vi "Get RGB Pixels Values.vi"(9 "I_Number of columns":i16, 10 "I_Number of rows":i16, 11 "I_Image Data":u8[](array[numeric])) -> (1 "O_RGB: Blue Color":u8[][](array[numeric]), 2 "O_RGB: Green Color":u8[][](array[numeric]), 3 "O_RGB: Red Color":u8[][](array[numeric]))   [LabVIEW 2015]
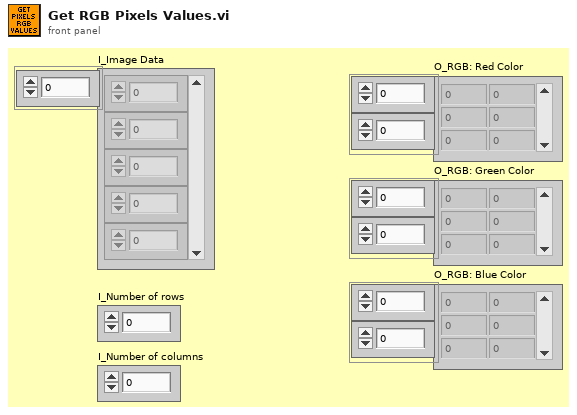
[diagram p1: front panel]
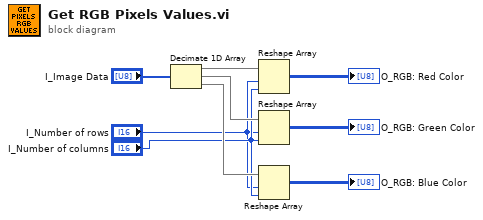
[diagram p0: block diagram]
diagram:
  n1 = Decimate 1D Array("I_Image Data") -> (w8:u8[], w7:u8[], w6:u8[])
  n2 = Reshape Array(w8, "I_Number of rows", "I_Number of columns") -> (→"O_RGB: Red Color":u8[][])
  n3 = Reshape Array(w7, "I_Number of rows", "I_Number of columns") -> (→"O_RGB: Green Color":u8[][])
  n4 = Reshape Array(w6, "I_Number of rows", "I_Number of columns") -> (→"O_RGB: Blue Color":u8[][])
